vi "Unpack Tree Double Click.vi"(0 "TreeDoubleClickMsg":refnum<class "TreeDoubleClickMsg.lvclass">) -> (3 "Control Label":string, 4 "CtlRef":refnum<vi>, 6 "Time":u32, 8 "Coords":T3, 10 "Button":u16, 12 "CellPart":T1(ring), 13 "Tag":string, 14 "PlatMods":T2, 15 "Mods":cluster{"Double Click":bool, "Menu Key":bool})   [LabVIEW 2017, in "ActorEvents.lvlib" / "TreeDoubleClickMsg.lvclass"]
doc: "<License>\nCopyright © 2017 Composed Systems, LLC | All rights reserved\nwww.composed.io\n\nAuthor: Ethan Stern <ethan.stern@composed.io>\n\nThis software is provided \"AS IS\" WITHOUT WARRANTIES, either express or implied, AND IS FOR EDUCATIONAL PURPOSES ONLY.\n</License>"
uses:
  TreeDoubleClickMsg.lvclass
  <vilib>/Utility/miscctls.llb/LVPoint32TypeDef.ctl
  TreeDoubleClickMsg.lvclass/TreeDoubleClickMsg.ctl
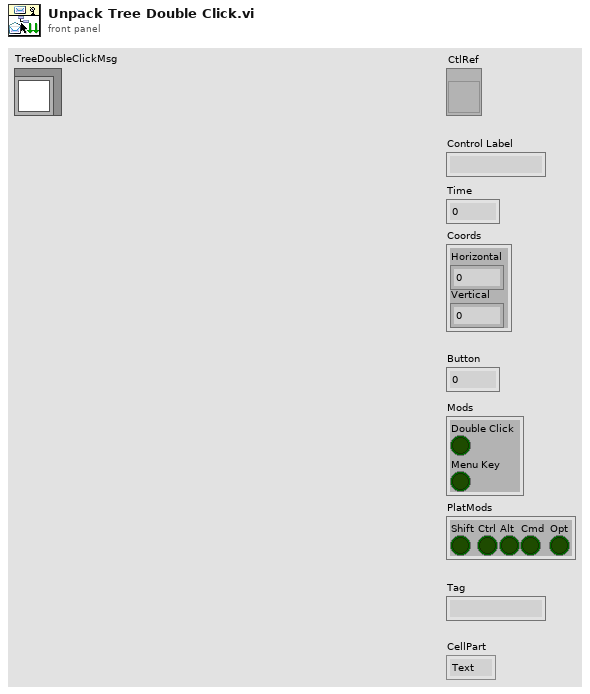
[diagram p1: front panel]
types:
  T1 = enum16{"Text", "Background", "Item Symbol", "Open/Close Symbol", "Hierarchy Lines", "Right Border", "Bottom Border", "Bottom Right Corner", "Unknown Part"}
  T2 = cluster{"Shift":bool, "Ctrl":bool, "Alt":bool, "Cmd":bool, "Opt":bool}
  T3 = typedef "LVPoint32TypeDef.ctl" = cluster{"Horizontal":i32, "Vertical":i32}
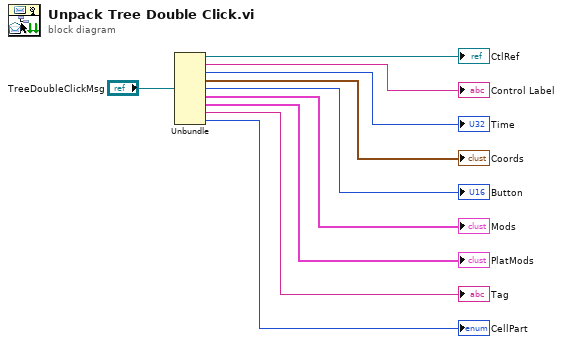
[diagram p0: block diagram]
diagram:
  n1 = Unbundle("TreeDoubleClickMsg") -> (→"CtlRef":refnum<vi>, →"Control Label":string, →"Time":u32, →"Coords":T3, →"Button":u16, →"Mods":cluster{"Double Click":bool, "Menu Key":bool}, →"PlatMods":T2, →"Tag":string, →"CellPart":T1)
